vi "Create Cursors.vi"(8 "Error In":errorcluster, 11 "Cursor List":T1) -> (0 "Error Out":errorcluster, 3 "Cursor List Out":T1)   [LabVIEW 2020]
uses:
  <vilib>/Utility/miscctls.llb/LVCursorListTypeDef.ctl
types:
  T1 = typedef "LVCursorListTypeDef.ctl" = cluster{"Name":string, "Color":u32, "Style":u8, "Point Style":u8, "Name Visible":bool, "Allow Drag":bool, "Cursor Mode":u32, "Plot":i32, "Index":i32, "Position":cluster{"X":dbl, "Y":dbl}, "X Scale":u32, "Y Scale":u32, "Watch Plots":i32[], "Watch All Plots":bool, "Plot Area":i32, "Label Offset":cluster{"X":dbl, "Y":dbl}}[]
  T2 = cluster{"Name":string, "Color":u32, "Style":u8, "Point Style":u8, "Name Visible":bool, "Allow Drag":bool, "Cursor Mode":u32, "Plot":i32, "Index":i32, "Position":cluster{"X":dbl, "Y":dbl}, "X Scale":u32, "Y Scale":u32, "Watch Plots":i32[], "Watch All Plots":bool, "Plot Area":i32, "Label Offset":cluster{"X":dbl, "Y":dbl}}
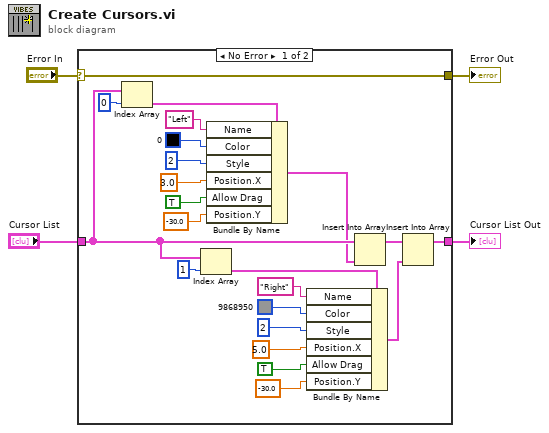
[diagram p0: block diagram]
diagram:
  n1 = case shown="No Error" "Error In" {
    selector: "Error In" -> [w7 w28]
    tunnel: [w7 w28] -> w3
    tunnel: "Cursor List" -> [w20 w27]
    tunnel: [w8 w27] -> w1
    frame No Error {
      n2 = Index Array(array=w20, index=0) -> (element=w24:T2)
      n3 = Index Array(array=w20, index=1) -> (element=w23:T2)
      n4 = Bundle By Name(cluster=w24, "Name"="Left", "Color"=u32 0, "Style"=u8 2, "Position.X"=3.0, "Allow Drag"=TRUE, "Position.Y"=-30.0) -> (w19:T2)
      n5 = Bundle By Name(cluster=w23, "Name"="Right", "Color"=u32 9868950, "Style"=u8 2, "Position.X"=5.0, "Allow Drag"=TRUE, "Position.Y"=-30.0) -> (w17:T2)
      n6 = Insert Into Array(array=w20, new element=w19) -> (w18:T1)  [unwired: 1 in]
      n7 = Insert Into Array(array=w18, new element=w17) -> (w8:T1)  [unwired: 1 in]
    }
    frame Error {
    }
  }
  "Error Out" <- w3
  "Cursor List Out" <- w1
